vi "Example Whlie Loop Some Operations 1.vi"(8 "Error In":errorcluster, 11 "Boolean":bool) -> (0 "Error Out":errorcluster, 3 "Numeric":i32)   [LabVIEW 2014]
doc: "Testing VI contains WhileLoop and som operations inside and some other constants and functions for numbers used inside WhileLoop. Just for example parsing."
uses:
  <vilib>/measure/NI_MABase.lvlib
panel:
  out "signal out 2":waveform(dbl)
  out "signal out":waveform(dbl)
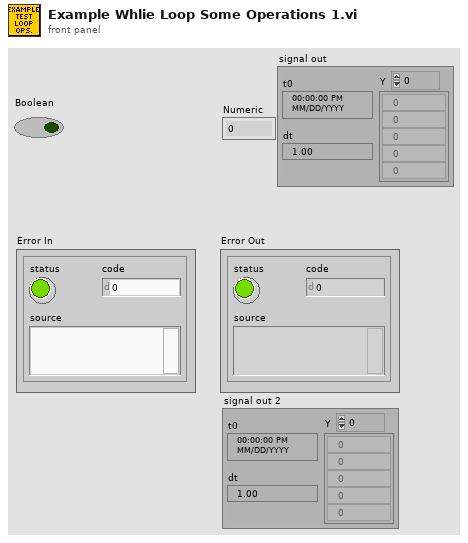
[diagram p1: front panel]
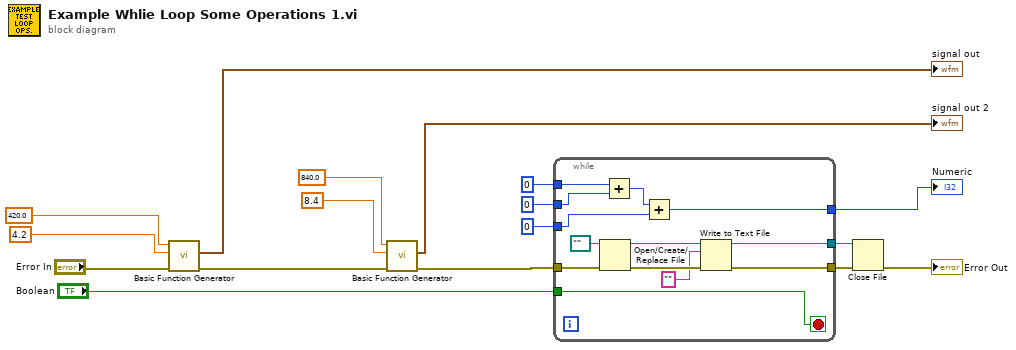
[diagram p0: block diagram]
diagram:
  n1 = call <vilib>:"Basic Function Generator.vi"("error in (no error)"="Error In", "amplitude"=4.2, "frequency"=420.0) -> ("error out"=w8:errorcluster, "signal out"=→"signal out":waveform(dbl))  [unwired: 6 in, 1 out]
  n2 = call <vilib>:"Basic Function Generator.vi"("error in (no error)"=w8, "amplitude"=8.4, "frequency"=840.0) -> ("error out"=w7:errorcluster, "signal out"=→"signal out 2":waveform(dbl))  [unwired: 6 in, 1 out]
  n3 = while {
    tunnel: 0 -> [w29]
    tunnel: 0 -> [w28]
    tunnel: 0 -> [w27]
    tunnel: "Boolean" -> [w26]
    tunnel: [w25] -> w13
    tunnel: w7 -> [w24]
    tunnel: [w23] -> w12
    tunnel: [w22] -> w10
    stop <- w26 stop-if-true
    n4 = Open/Create/Replace File(file path (use dialog)=path "", error in=w24) -> (refnum out=w21:refnum<file>, error out=w19:errorcluster)  [unwired: 4 in, 1 out]
    n5 = Add(x=w29, y=w28) -> (x+y=w30:i32)
    n6 = Add(x=w30, y=w27) -> (x+y=w25:i32)
    n7 = Write to Text File(file (use dialog)=w21, text="", error in=w19) -> (refnum out=w22:refnum<file>, error out=w23:errorcluster)  [unwired: 1 in, 1 out]
  }
  "Numeric" <- w13
  n8 = Close File(refnum=w10, error in=w12) -> (error out=→"Error Out":errorcluster)  [unwired: 1 out]
